vi "Light Control.vi"() -> ()   [LabVIEW 2013]
uses:
  <vilib>/Instr/_visa.llb/VISA Configure Serial Port (Instr).vi
panel:
  in  "Stop":bool
  out "error out":errorcluster
  in  "error in (no error)":errorcluster
  in  "Light Value":i32(slide) scale=0.0..255.0
  in  "Light COM Port":refnum<visa-resource-name>
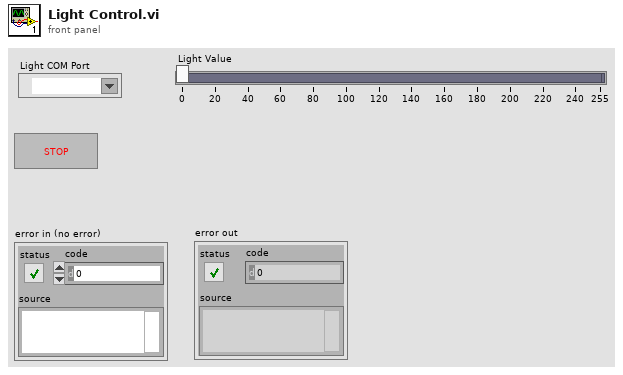
[diagram p1: front panel]
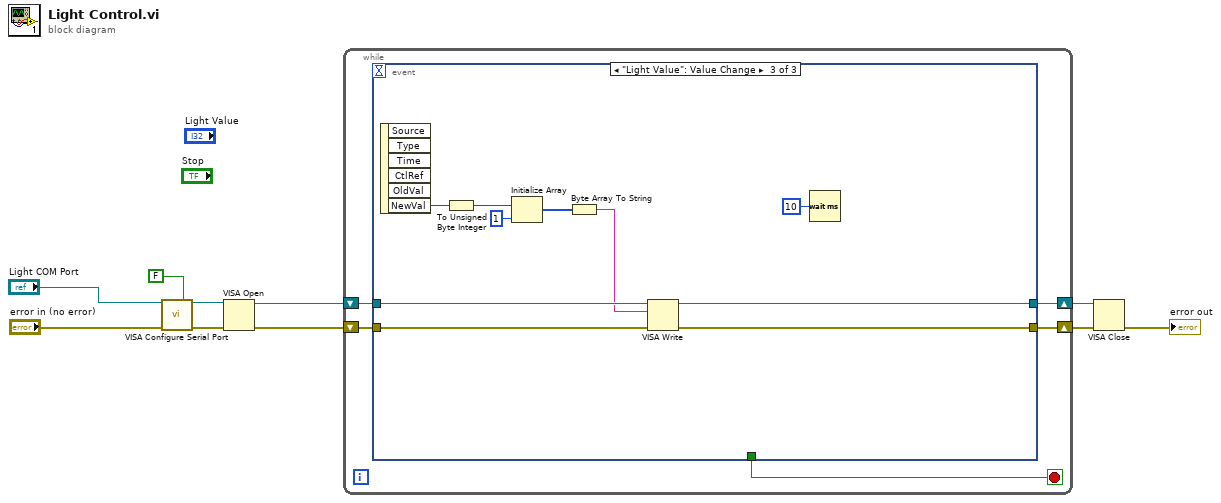
[diagram p0: block diagram]
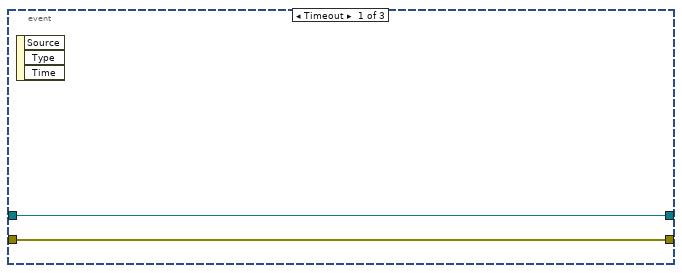
[diagram p2: hidden frame]
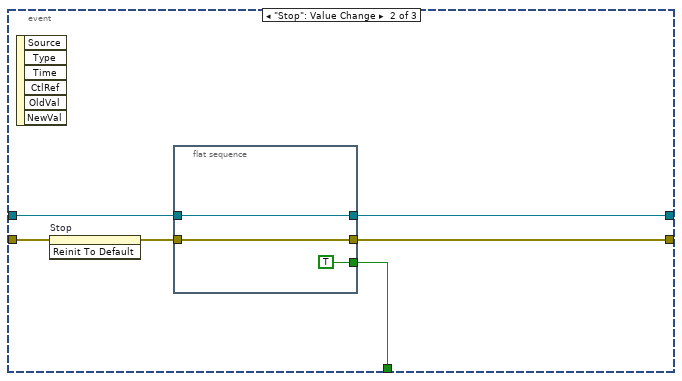
[diagram p3: hidden frame]
diagram:
  n1 = call-poly "VISA Configure Serial Port"("VISA resource name"="Light COM Port", "Enable Termination\nChar (T)"=FALSE ("Enable Termination\nChar (T)"), "error in (no error)"="error in (no error)") -> ("VISA resource name out"=w6:refnum<visa-resource-name>, "error out"=w7:errorcluster)  [unwired: 11 in]
  n2 = VISA Open(error in (no error)=w7, VISA resource name=w6) -> (VISA resource name=w5:refnum<visa-resource-name>, error out=w4:errorcluster)  [unwired: 3 in]
  n3 = while {
    shift-right: [w14] -> w3
    shift-left: w4 -> [w15]
    shift-right: [w11] -> w2
    shift-left: w5 -> [w12]
    stop <- w13 stop-if-true
    n4 = event shown="[2] \"Light Value\": Value Change" {
      selector: _ -> [_ _ _]
      dyn-events: _ -> [_ _ _]
      timeout: _ -> [_ _ _]
      tunnel: w15 -> [w17 w23 w36]
      tunnel: [w17 w21 w34] -> w14
      tunnel: [_ w20 _] -> w13
      tunnel: w12 -> [w16 w19 w35]
      tunnel: [w16 w18 w33] -> w11
      event Timeout {
        n5 = event-data() -> ()  [unwired: 1 in, 3 out]
      }
      event "Stop": Value Change {
        n6 = event-data() -> ()  [unwired: 1 in, 6 out]
        n7 = invoke on="Stop" class="Bool" method="Reinit To Default"(error in=w23) -> (error out=w22:errorcluster)  [unwired: 2 in, 2 out]
        n8 = flat-sequence {
          tunnel: w22 -> [w26]
          tunnel: [w26] -> w21
          tunnel: [TRUE] -> w20
          tunnel: w19 -> [w24]
          tunnel: [w24] -> w18
          frame #0 {
          }
        }
      }
      event "Light Value": Value Change {
        n9 = event-data() -> ("NewVal"=w31:i32)  [unwired: 1 in, 5 out]
        n10 = To Unsigned Byte Integer(number=w31) -> (unsigned 8bit integer=w30:u8)
        n11 = Initialize Array(w30, 1 ("dimension size")) -> (w28:u8[])
        n12 = Byte Array To String(unsigned byte array=w28) -> (string=w27:string)
        n13 = VISA Write(VISA resource name=w35, write buffer=w27, error in (no error)=w36) -> (VISA resource name out=w33:refnum<visa-resource-name>, error out=w34:errorcluster)  [unwired: 1 out]
        n14 = Wait (ms)(milliseconds to wait=u32 10) -> ()  [unwired: 1 out]
      }
    }
  }
  n15 = VISA Close(VISA resource name=w2, error in (no error)=w3) -> (error out=→"error out":errorcluster)
